vi "addVoxelsToLines.vi"(8 "error in":errorcluster, 9 "idle?":bool, 10 "Queues":T2, 11 "FPGA VI ref":T1) -> (0 "error out":errorcluster, 2 "num elements available":u32, 3 "num zero volume lines":u32, 4 "num elements requested":u32, 5 "lines with no data":i32, 6 "num read":u32, 7 "lines read":u32)   [LabVIEW 2010]
uses:
  internal_queues.ctl
  line_info.ctl
  volume_with_lines.ctl
  volume_info.ctl
  kalman_result_scaled.ctl
  projection buffers.ctl
  location3D.ctl
  spot location.ctl
  FPGA_ref.ctl
  <vilib>/rvi/interface/nirviMethod/nirviMethod.xnode
  <vilib>/rvi/interface/common/niFpgaNodeNameForErrorReporting.ctl
  <vilib>/rvi/errors/niLvFpgaWhatHappensToTopLevelVI.ctl
  <vilib>/rvi/interface/nirviReadWriteControl/nirviReadWriteControl.xnode
  <vilib>/Utility/error.llb/Error Cluster From Error Code.vi
  <vilib>/rvi/errors/niLvFpgaAdjustHostInterfaceError.vi
  NiFpgaLv.dll
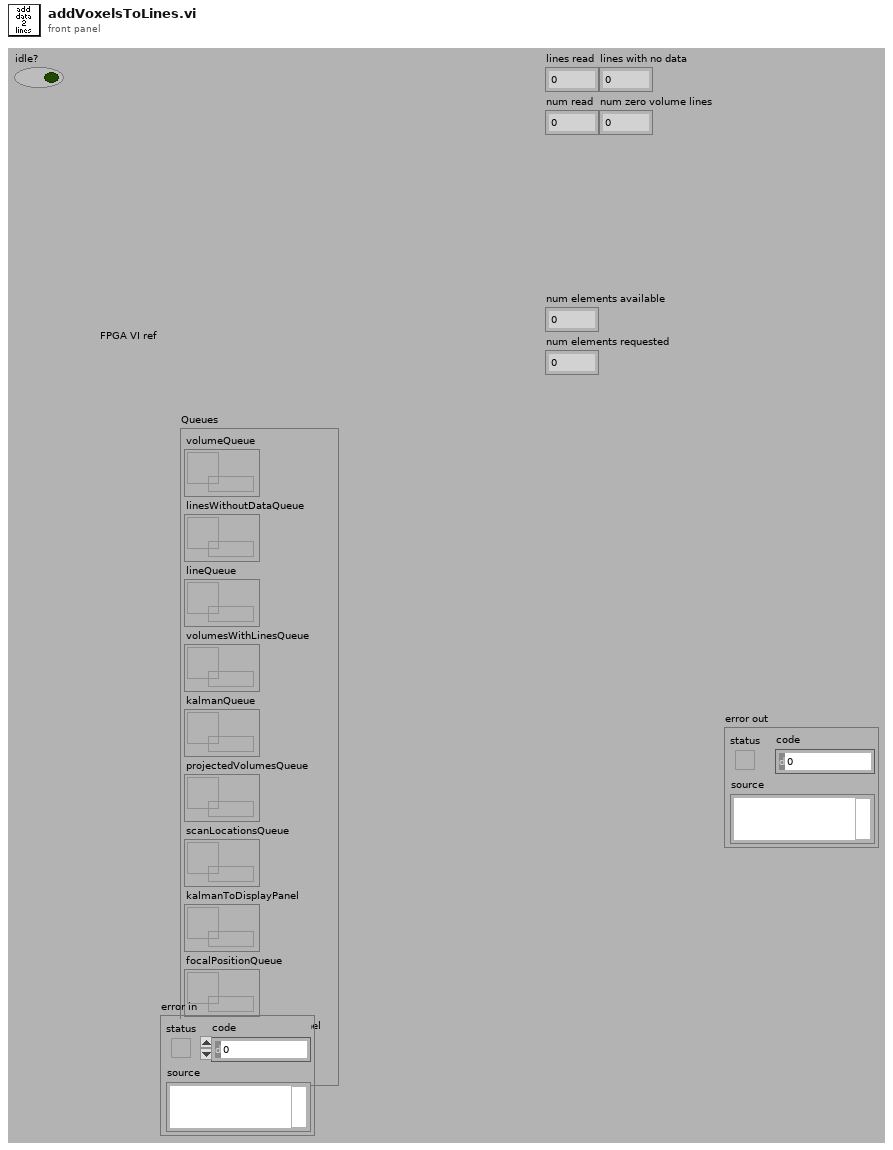
[diagram p1: front panel]
types:
  T1 = typedef "FPGA_ref.ctl" = refnum<k20>
  T2 = typedef "internal_queues.ctl" = cluster{"volumeQueue":refnum<queue>, "linesWithoutDataQueue":refnum<queue>, "lineQueue":refnum<queue>, "volumesWithLinesQueue":refnum<queue>, "kalmanQueue":refnum<queue>, "projectedVolumesQueue":refnum<queue>, "scanLocationsQueue":refnum<queue>, "kalmanToDisplayPanel":refnum<queue>, "focalPositionQueue":refnum<queue>, "spotPositionsToImagePanel":refnum<queue>}
  T3 = typedef "niFpgaNodeNameForErrorReporting.ctl" = enum16{"Open FPGA VI Reference", "Read/Write Control", "Invoke Method: Abort", "Invoke Method: Acknowledge IRQ", "Invoke Method: Download", "Invoke Method: FIFO.Configure", "Invoke Method: FIFO.Read", "Invoke Method: FIFO.Start", "Invoke Method: FIFO.Stop", "Invoke Method: FIFO.Write", "Invoke Method: Reset", "Invoke Method: Run", "Invoke Method: Wait on IRQ", "Close FPGA VI Reference"}
  T4 = typedef "niLvFpgaWhatHappensToTopLevelVI.ctl" = enum16{"top level VI scripted behind XNode", "top level VI inlined behind XNode"}
  T5 = typedef "line_info.ctl" = cluster{"start X":i16, "start Y":i16, "start Z":i16, "end X":i16, "end Y":i16, "end Z":i16, "num z":u8, "voxel data":u32[], "volume num":u32, "line number":u16, "line type":u16}
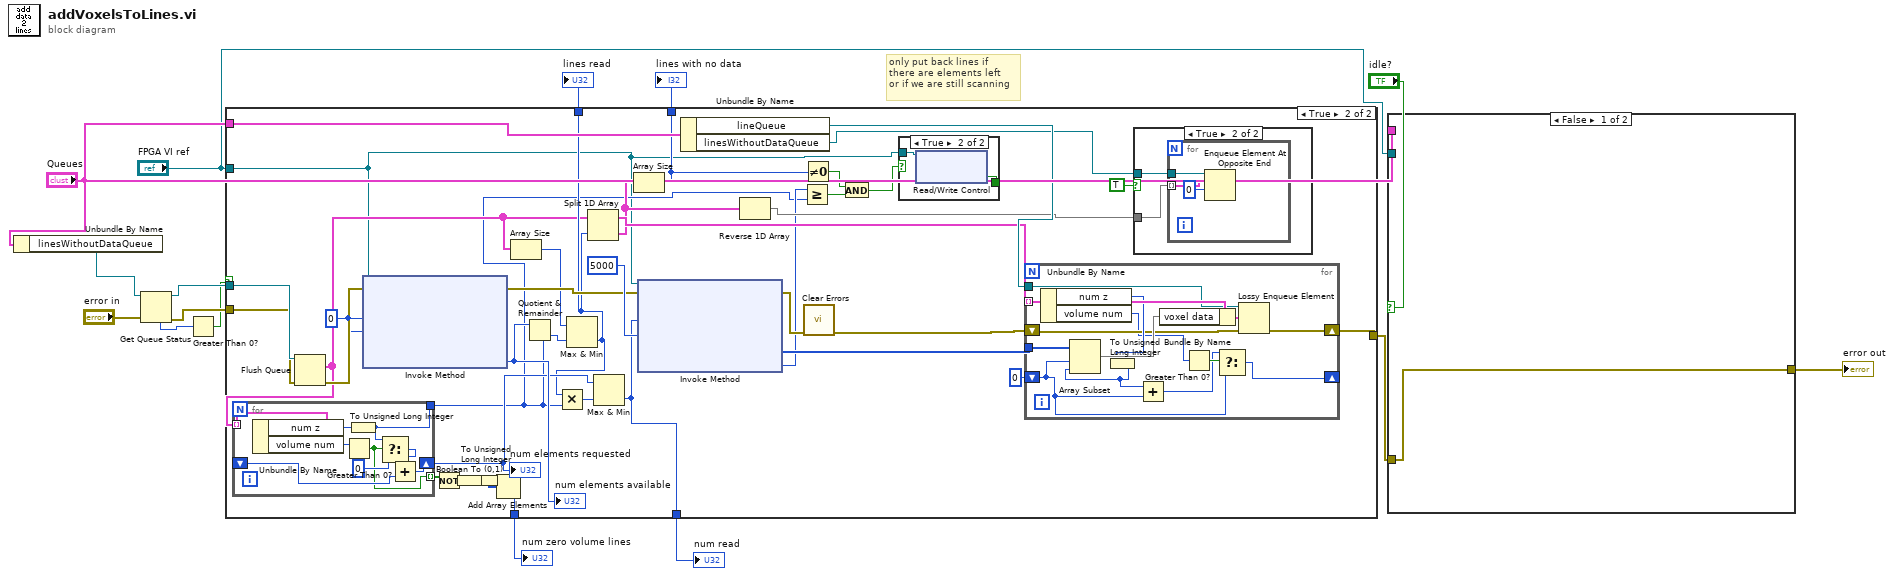
[diagram p0: block diagram]
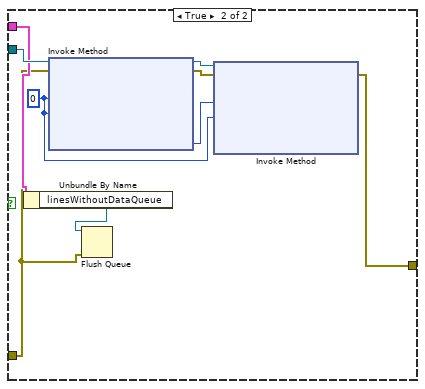
[diagram p2: hidden frame]
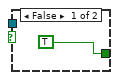
[diagram p4: hidden frame]
diagram:
  # "only put back lines if\nthere are elements left\nor if we are still scanning"
  n1 = Unbundle By Name("Queues") -> ("linesWithoutDataQueue"=w15:refnum<queue>)
  n2 = Get Queue Status(queue=w15, error in (no error)="error in") -> (queue out=w13:refnum<queue>, error out=w12:errorcluster, # elements in queue=w14:i32)  [unwired: 1 in, 5 out]
  n3 = Greater Than 0?(x=w14) -> (x > 0?=w10:bool)
  n4 = case shown="True" w10 {
    tunnel: "Queues" -> [_ w37]
    tunnel: w13 -> [_ w51]
    tunnel: w12 -> [w16 w50]
    tunnel: [w16 w49] -> w4
    tunnel: [_ w35] -> w9
    tunnel: [_ w31] -> w8
    tunnel: [_ w20] -> w7
    tunnel: [_ w19] -> w6
    tunnel: "FPGA VI ref" -> [_ w18]
    frame False {
    }
    frame True {
      w47 = u32 0 ("Number of Elements")
      n5 = Flush Queue(queue=w51, error in (no error)=w50) -> (remaining elements=w34:T5[], error out=w48:errorcluster)  [unwired: 1 out]
      n6 = for {
        tunnel: w34 -> [w114] mode=indexing
        shift-right: [w113] -> w36
        shift-left: _ -> [w108]
        tunnel: [w107] -> w26
        tunnel: [w106] -> w24 mode=indexing
        n7 = Unbundle By Name(w114) -> ("num z"=w111:u8, "volume num"=w112:u32)
        n8 = Greater Than 0?(x=w112) -> (x > 0?=w106:bool)
        n9 = To Unsigned Long Integer(number=w111) -> (unsigned 32bit integer=w107:u32)
        n10 = Select(t=w107, s=w106, f=u32 0) -> (s? t:f=w109:u32)
        n11 = Add(x=w109, y=w108) -> (x+y=w113:u32)
      }
      "num elements requested" <- w36
      n12 = xnode "Invoke Method"("FPGA VI Reference In"=w18, "error in"=w48, "Number of Elements"=w47, "Timeout (ms)"=w47) -> ("error out"=w41:errorcluster, "Elements Remaining"=w46:u32)  [unwired: 2 out]
      "num elements available" <- w46
      n13 = Not(x=w24) -> (.not. x?=w22:bool[])
      n14 = Boolean To (0,1)(Boolean=w22) -> (0, 1=w23:i16[])
      n15 = To Unsigned Long Integer(number=w23) -> (unsigned 32bit integer=w21:u32[])
      n16 = Add Array Elements(numeric array=w21) -> (sum=w19:u32)
      n17 = Array Size(array=w34) -> (size(s)=w33:i32)
      n18 = Quotient & Remainder(x=w46, y=w26) -> (floor(x/y)=w32:u32)  [unwired: 1 out]
      n19 = Max & Min(x=w33, y=w32) -> (min(x,y)=w35:u32)  [unwired: 1 out]
      n20 = Multiply(x=w35, y=w26) -> (x*y=w45:u32)
      n21 = Split 1D Array(array=w34, index=w35) -> (first subarray=w44:T5[], second subarray=w40:T5[])
      n22 = Max & Min(x=w36, y=w45) -> (min(x,y)=w20:u32)  [unwired: 1 out]
      n23 = Array Size(array=w40) -> (size(s)=w31:i32)
      n24 = xnode "Invoke Method"("FPGA VI Reference In"=w18, "error in"=w41, "Number of Elements"=w20, "Timeout (ms)"=5000) -> ("error out"=w38:errorcluster, "Data"=w39:u32[], "Elements Remaining"=w27:u32)  [unwired: 1 out]
      n25 = Unbundle By Name(w37) -> ("lineQueue"=w54:refnum<queue>, "linesWithoutDataQueue"=w42:refnum<queue>)
      n26 = Reverse 1D Array(array=w40) -> (reversed array=w43:T5[])
      n27 = Greater Or Equal?(x=w27, y=w26) -> (x >= y?=w30:bool)
      n28 = Not Equal To 0?(x=w31) -> (x != 0?=w29:bool)
      n29 = call <vilib>:"Clear Errors.vi"("error in (no error)"=w38) -> ("error out"=w17:errorcluster)  [unwired: 6 in]
      n30 = And(x=w29, y=w30) -> (x .and. y?=w28:bool)
      n31 = case shown="True" w28 {
        tunnel: w18 -> [_ w57]
        tunnel: [TRUE ("scanning?") w56] -> _
        frame False {
        }
        frame True {
          n32 = xnode "Read/Write Control"("FPGA VI Reference In"=w57) -> ("scanning?"=w56:bool)  [unwired: 1 in, 2 out]
        }
      }
      n33 = for {
        tunnel: w44 -> [w200] mode=indexing
        tunnel: w39 -> [w201]
        shift-right: [w189] -> _
        shift-left: u32 0 -> [w190]
        shift-right: [w194] -> w49
        shift-left: w17 -> [w195]
        tunnel: w54 -> [w196]
        n34 = Unbundle By Name(w200) -> ("num z"=w198:u8, "volume num"=w193:u32)
        n35 = To Unsigned Long Integer(number=w198) -> (unsigned 32bit integer=w188:u32)
        n36 = Array Subset(array=w201, index=w190, length=w188) -> (w199:u32[])
        n37 = Add(x=w188, y=w190) -> (x+y=w191:u32)
        n38 = Bundle By Name(cluster=w200, "voxel data"=w199) -> (w197:T5)
        n39 = Greater Than 0?(x=w193) -> (x > 0?=w192:bool)
        n40 = Select(t=w191, s=w192, f=w190) -> (s? t:f=w189:u32)
        n41 = Lossy Enqueue Element(queue=w196, element=w197, error in (no error)=w195) -> (error out=w194:errorcluster)  [unwired: 3 out]
      }
      n42 = case shown="True" TRUE {
        tunnel: w43 -> [_ w102]
        tunnel: w42 -> [_ w101]
        frame False {
        }
        frame True {
          n43 = for {
            tunnel: w102 -> [w105] mode=indexing
            tunnel: w101 -> [w104]
            n44 = Enqueue Element At Opposite End(queue=w104, element=w105, timeout in ms (-1)=0) -> ()  [unwired: 1 in, 3 out]
          }
        }
      }
    }
  }
  "lines read" <- w9
  "lines with no data" <- w8
  "num read" <- w7
  "num zero volume lines" <- w6
  n45 = case shown="False" "idle?" {
    tunnel: w4 -> [w275 w277]
    tunnel: "Queues" -> [_ w279]
    tunnel: "FPGA VI ref" -> [_ w284]
    tunnel: [w275 w276] -> w1
    frame False {
    }
    frame True {
      w282 = u32 0 ("Number of Elements")
      n46 = Unbundle By Name(w279) -> ("linesWithoutDataQueue"=w278:refnum<queue>)
      n47 = xnode "Invoke Method"("FPGA VI Reference In"=w284, "error in"=w277, "Number of Elements"=w282, "Timeout (ms)"=w282) -> ("FPGA VI Reference Out"=w280:T1, "error out"=w281:errorcluster, "Elements Remaining"=w283:u32)  [unwired: 1 out]
      n48 = Flush Queue(queue=w278, error in (no error)=w277) -> ()  [unwired: 3 out]
      n49 = xnode "Invoke Method"("FPGA VI Reference In"=w280, "error in"=w281, "Number of Elements"=w283, "Timeout (ms)"=w282) -> ("error out"=w276:errorcluster)  [unwired: 3 out]
    }
  }
  "error out" <- w1
